vi "WPI_CameraClose Internal.vi"(8 "error in (no error)":errorcluster, 11 "CameraDevRef":T1) -> (0 "error out":errorcluster)   [LabVIEW 2017]
doc: "This software is licensed. Open the labview\\readme\\WPI Robotics Library Open Source License.txt file for more information."
uses:
  <vilib>/Rock Robotics/WPI/Camera/WPI_CameraDevRef.ctl
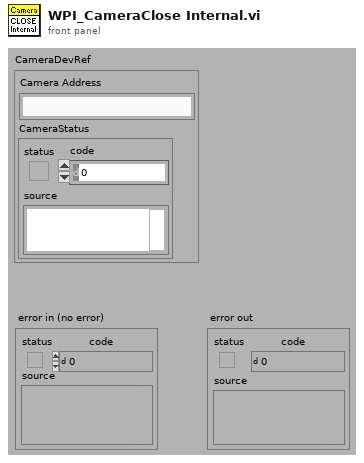
[diagram p1: front panel]
types:
  T1 = typedef "WPI_CameraDevRef.ctl" = cluster{"Camera Address":string, "CameraStatus":errorcluster}
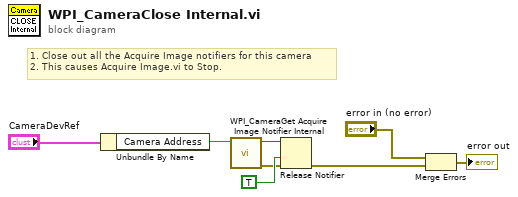
[diagram p0: block diagram]
diagram:
  # "1. Close out all the Acquire Image notifiers for this camera\n2. This causes Acquire Image.vi to Stop."
  n1 = Unbundle By Name("CameraDevRef") -> ("Camera Address"=w5:string)
  n2 = call <vilib>:"WPI_CameraGet Acquire Image Notifier Internal.vi"("Camera Address"=w5) -> ("error out"=w1:errorcluster, "Acquire Image Notifier"=w2:refnum<notifier>)  [unwired: 1 in, 8 out]
  n3 = Release Notifier(notifier=w2, force destroy? (F)=TRUE, error in (no error)=w1) -> (error out=w4:errorcluster)  [unwired: 2 out]
  n4 = Merge Errors("error in (no error)", w4) -> (→"error out":errorcluster)
